vi "Alphabetize.vi"(8 "Error In":errorcluster) -> (0 "Error Out":errorcluster)   [LabVIEW 2017, in "Tests.lvlib" / "Toolkit.lvlib"]
uses:
  Toolkit.lvlib
  <vilib>/Utility/traverseref.llb/TRef TravTarget.ctl
  Support VIs/Alphabetize Target.vi
  <vilib>/addons/_JKI Toolkits/Caraya/classes/Test/Test.lvclass
  src/Toolkit/Toolkit.lvlib
  <vilib>/Utility/traverseref.llb/VI Scripting - Traverse.lvlib
  <vilib>/addons/_JKI Toolkits/Caraya/classes/Assert/Assert.lvclass
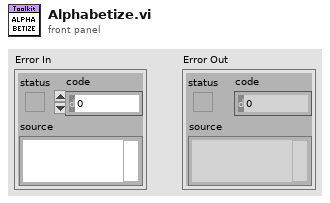
[diagram p1: front panel]
types:
  T1 = typedef "TRef TravTarget.ctl" = enum16{"FP", "BD", "Other"}
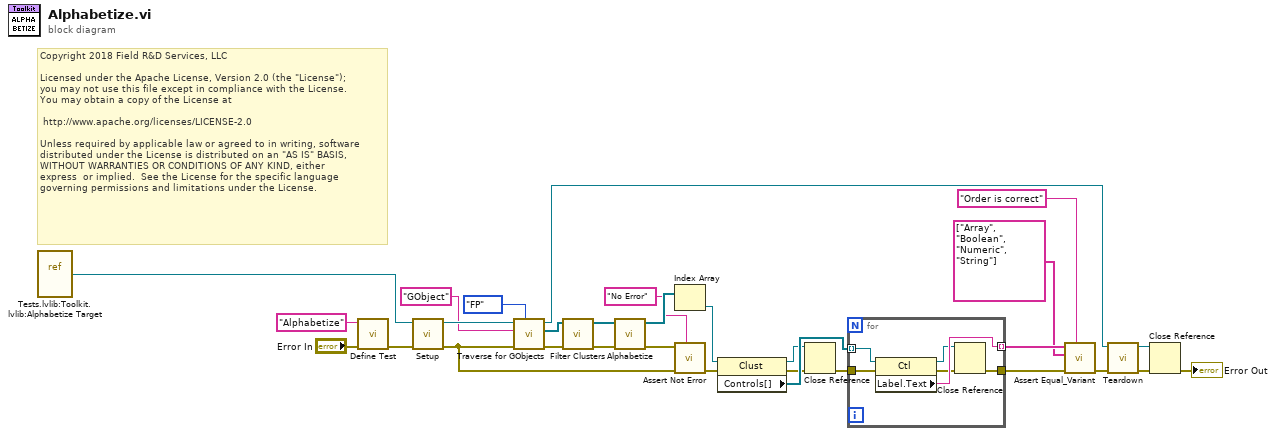
[diagram p0: block diagram]
diagram:
  # "Copyright 2018 Field R&D Services, LLC\n\nLicensed under the Apache License, Version 2.0 (the \"License\");\nyou may not use this file except in compliance with the License.\nYou may obtain a copy of the License at\n\n\thttp://www.apache.org/licenses/LICENSE-2.0\n\nUnless required by applicable law or agreed to in writing, software\ndistributed under the License is distributed on an \"AS IS\" BASIS,\nWITHOUT WARRANTIES OR CONDITIONS OF ANY KIND, either \nexpress  or implied.  See the License for the specific language \ngoverning permissions and limitations under the License."
  n1 = vi-ref "Tests.lvlib:Toolkit.lvlib:Alphabetize Target.vi"() -> (w27:refnum<vi>)
  n2 = call <vilib>:"Define Test.vi"("error in (no error)"="Error In", "Label (VI Title)"="Alphabetize") -> ("error out"=w28:errorcluster)  [unwired: 9 in]
  n3 = call "Setup.vi"("Error In"=w28, "VI In"=w27) -> ("Error Out"=w6:errorcluster, "VI Out"=w25:refnum<vi>)  [unwired: 8 in]
  n4 = call <vilib>:"Traverse for GObjects.vi"("Traverse Target"=TRef_TravTarget."FP", "error in (no error)"=w6, "Class Name"="GObject", "VI Refnum"=w25) -> ("error out"=w22:errorcluster, "References"=w23:refnum<vi>[], "dup VI Refnum"=w4:refnum<vi>)  [unwired: 4 in, 1 out]
  n5 = call "Filter Clusters.vi"("Error In"=w22, "GObjects"=w23) -> ("Error Out"=w21:errorcluster, "Clusters"=w20:refnum<vi>[])  [unwired: 8 in]
  n6 = call "Alphabetize.vi"("Error In"=w21, "Clusters In"=w20) -> ("Error Out"=w9:errorcluster, "Clusters Out"=w17:refnum<vi>[])  [unwired: 8 in]
  n7 = Index Array(array=w17) -> (element=w16:refnum<vi>)  [unwired: 1 in]
  n8 = call <vilib>:"Assert Not Error.vi"("Label"="No Error", "error in (no error)"=w6, "Not Error?"=w9) -> ("error out"=w8:errorcluster)  [unwired: 8 in]
  n9 = property class="Clust"(reference=w16, error in=w8) -> (reference out=w14:refnum<vi>, error out=w18:errorcluster, "Controls[]"=w19:refnum<vi>[])
  n10 = Close Reference(reference=w14, error in (no error)=w18) -> (error out=w15:errorcluster)
  n11 = for {
    tunnel: w19 -> [w36] mode=indexing
    tunnel: w15 -> [w35]
    tunnel: [w34] -> w13 mode=indexing
    tunnel: [w31] -> w7
    n12 = property class="Ctl"(reference=w36, error in=w35) -> (reference out=w32:refnum<vi>, error out=w33:errorcluster, "Label.Text"=w34:string)
    n13 = Close Reference(reference=w32, error in (no error)=w33) -> (error out=w31:errorcluster)
  }
  n14 = call <vilib>:"Assert Equal_Variant.vi"("Label"="Order is correct", "error in (no error)"=w7, "Y"=string[] ["Array", "Boolean", "Numeric", "String"], "X"=w13) -> ("error out"=w5:errorcluster)  [unwired: 7 in]
  n15 = call "Teardown.vi"("Error In"=w5, "VI In"=w4) -> ("Error Out"=w2:errorcluster, "VI Out"=w3:refnum<vi>)  [unwired: 8 in]
  n16 = Close Reference(reference=w3, error in (no error)=w2) -> (error out=→"Error Out":errorcluster)
